vi "Get Section.vi"(8 "sections":string[](array[string]), 11 "info data":string) -> (0 "sections out":string[](array[string]), 1 "exist":bool, 3 "section part":string)   [LabVIEW 2019, in "infolib.lvlib"]
doc: "Finds section structure and return its content. If not found, exist is false. If no section structure set, returns whole info data and exist is true."
uses:
  infolib.lvlib
  <vilib>/Utility/error.llb/whitespace.ctl
  <vilib>/regexp/Match Regular Expression.xnode
panel:
  # "testing string: (put \"1\" and \"2\" into section names)"
  # "blfdablad\n#startsection:: 1\njfkdla\n#startsection:: 2\ngroup2group2\n\t  \t#endsection:: 2\njdfkls\n#endsection:: 1\njfdklajfkdl"
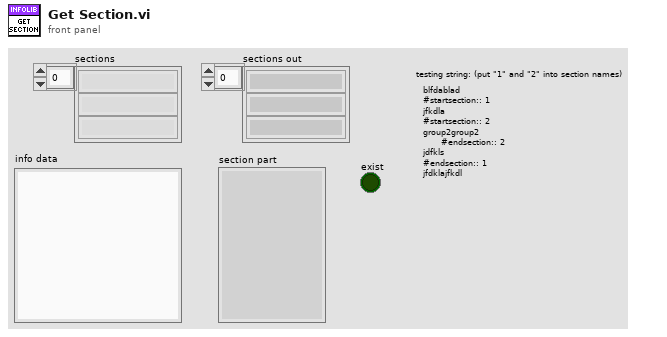
[diagram p1: front panel]
types:
  T1 = typedef "whitespace.ctl" = u16
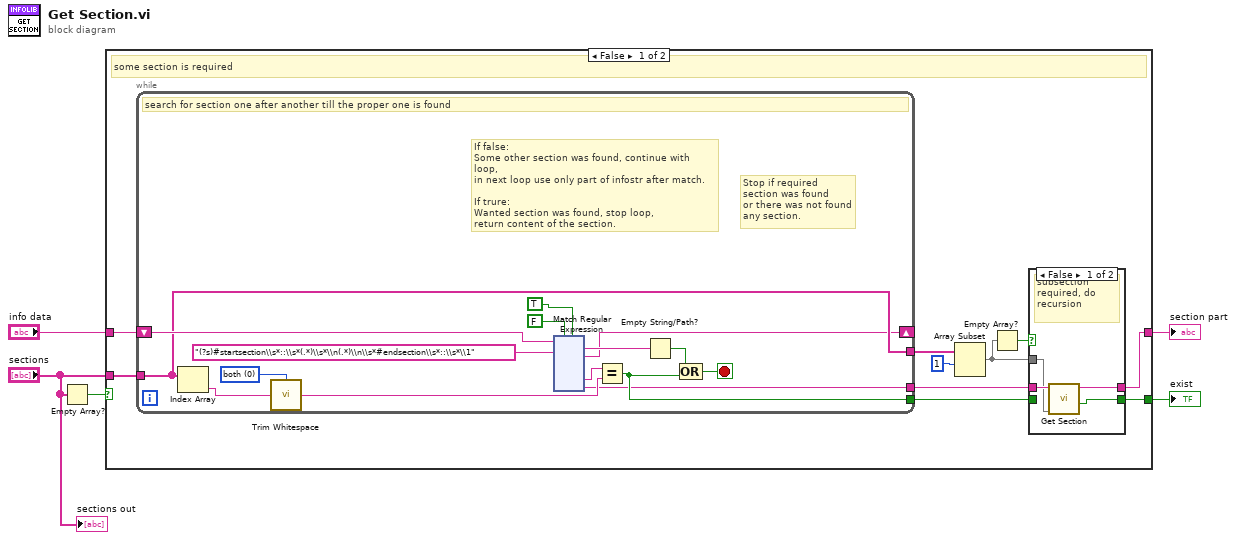
[diagram p0: block diagram]
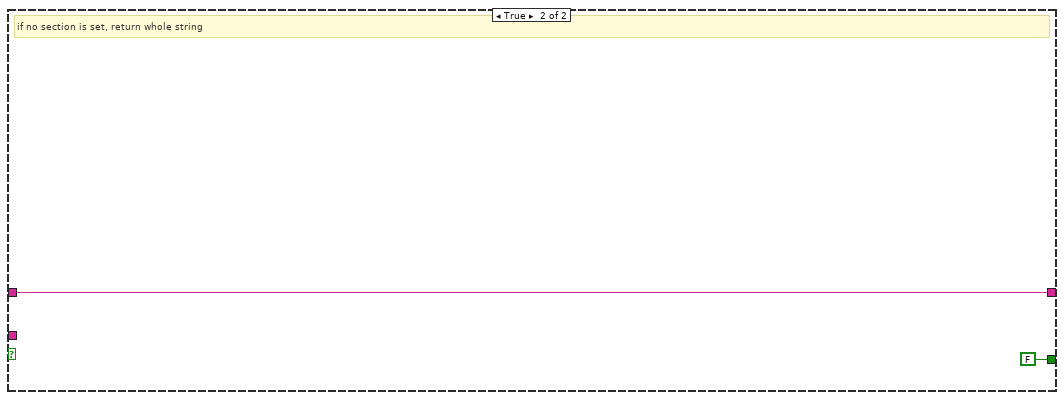
[diagram p3: hidden frame]
diagram:
  n1 = Empty Array?(array="sections") -> (empty?=w5:bool)
  n2 = case shown="False" w5 {
    tunnel: "sections" -> [w15 _]
    tunnel: "info data" -> [w14 w154]
    tunnel: [w8 w154] -> w2
    tunnel: [w7 FALSE ("exist")] -> w1
    frame False {
      # "some section is required"
      n3 = while {
        tunnel: w15 -> [w28]
        tunnel: [w22] -> w10
        shift-right: [w24] -> _
        shift-left: w14 -> [w33]
        tunnel: [w28] -> w12
        tunnel: [w23] -> w6
        stop <- w29 stop-if-true
        w27 = T1 0 items=["both", "start of string", "end of string"] ("location (both)")
        # "Stop if required\nsection was found\nor there was not found\nany section."
        # "If false:\nSome other section was found, continue with loop,\nin next loop use only part of infostr after match.\n\nIf trure:\nWanted section was found, stop loop,\nreturn content of the section."
        # "search for section one after another till the proper one is found"
        n4 = Index Array(array=w28) -> (element=w26:string)  [unwired: 1 in]
        n5 = call <vilib>:"Trim Whitespace.vi"("string"=w26, "location (both)"=w27) -> ("trimmed string"=w25:string)
        n6 = xnode "Match Regular Expression"("input string"=w33, "regular expression"="(?s)#startsection\\s*::\\s*(.*)\\s*\\n(.*)\\n\\s*#endsection\\s*::\\s*\\1" ("format string"), "ignore case? (F)"=FALSE, "multiline? (F)"=TRUE) -> ("whole match"=w32:string, "after match"=w24:string, "submatch 1"=w31:string, "submatch 2"=w22:string)  [unwired: 2 in, 3 out]
        n7 = Equal?(x=w31, y=w25) -> (x = y?=w23:bool)
        n8 = Empty String/Path?(string/path=w32) -> (empty?=w30:bool)
        n9 = Compound Arithmetic op=OR(w30, w23) -> (w29:bool)
      }
      n10 = Array Subset(array=w12, index=1) -> (w11:string[])  [unwired: 1 in]
      n11 = Empty Array?(array=w11) -> (empty?=w9:bool)
      n12 = case shown="False" w9 {
        tunnel: w10 -> [w19 w21]
        tunnel: [w18 w21] -> w8
        tunnel: w11 -> [w17 _]
        tunnel: [w16 w20] -> w7
        tunnel: w6 -> [_ w20]
        frame False {
          # "subsection\nrequired, do\nrecursion"
          n13 = call "Get Section.vi"("sections"=w17, "info data"=w19) -> ("exist"=w16:bool, "section part"=w18:string)  [unwired: 7 in, 1 out]
        }
        frame True {
          # "subsection not\nrequired"
        }
      }
    }
    frame True {
      # "if no section is set, return whole string"
    }
  }
  "exist" <- w1
  "section part" <- w2
  "sections out" <- "sections"
